vi "EI1050 Read.vi"(8 "error in":errorcluster, 10 "Enable Channel (or -1)":i32=3, 11 "Handle In":i32) -> (0 "error out":errorcluster, 1 "RH [%]":dbl format="%.6f", 2 "Temp [degC]":dbl format="%.6f", 3 "Handle Out":i32, 4 "Temp [degF]":dbl format="%.6f")   [LabVIEW 2021]
panel:
  # "Pass -1 if not using enable/disable."
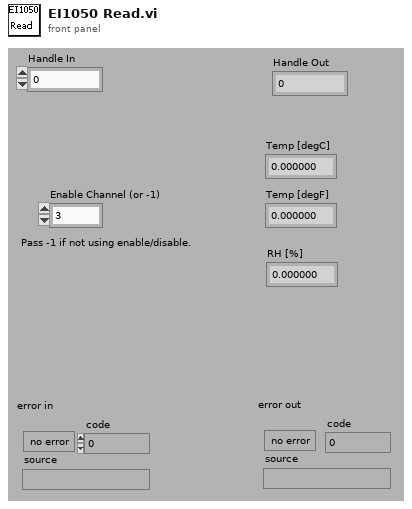
[diagram p1: front panel]
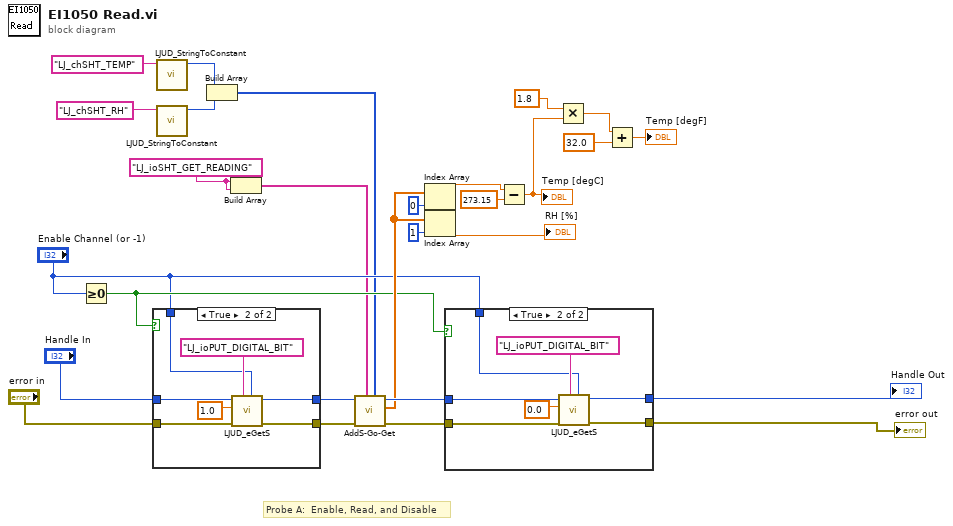
[diagram p0: block diagram]
diagram:
  w12 = "LJ_ioSHT_GET_READING" ("IOType")
  # "Probe A:  Enable, Read, and Disable"
  n1 = Greater Or Equal To 0?(x="Enable Channel (or -1)") -> (x >= 0?=w16:bool)
  n2 = case shown="True" w16 {
    tunnel: [w29 w37] -> w26
    tunnel: [w30 w36] -> w25
    tunnel: "error in" -> [w29 w33]
    tunnel: "Handle In" -> [w30 w32]
    tunnel: "Enable Channel (or -1)" -> [_ w31]
    frame False {
    }
    frame True {
      n3 = call "LJUD_eGetS.vi"("Channel"=w31, "IOType"="LJ_ioPUT_DIGITAL_BIT", "error in"=w33, "Value Write"=1.0, "Handle In"=w32) -> ("error out"=w37:errorcluster, "Handle Out"=w36:i32)  [unwired: 4 in, 1 out]
    }
  }
  n4 = call "LJUD_StringToConstant.vi"("String"="LJ_chSHT_TEMP") -> ("Constant Number"=w11:i32)  [unwired: 9 in, 1 out]
  n5 = call "LJUD_StringToConstant.vi"("String"="LJ_chSHT_RH") -> ("Constant Number"=w10:i32)  [unwired: 9 in, 1 out]
  n6 = Build Array(w11, w10) -> (w6:i32[])
  n7 = Build Array(w12, w12) -> (w7:string[])
  n8 = call "AddS-Go-Get.vi"("Channels"=w6, "IOTypes"=w7, "error in"=w26, "Handle In"=w25) -> ("error out"=w28:errorcluster, "Values Read"=w22:dbl[], "Handle Out"=w27:i32)  [unwired: 5 in]
  n9 = Index Array(array=w22, index=0 ("Index")) -> (element=w24:dbl)
  n10 = Index Array(array=w22, index=1 ("Index")) -> (element=→"RH [%]":dbl)
  n11 = case shown="True" w16 {
    tunnel: w28 -> [w38 w46]
    tunnel: w27 -> [w39 w45]
    tunnel: "Enable Channel (or -1)" -> [_ w42]
    tunnel: [w38 w41] -> w14
    tunnel: [w39 w40] -> w13
    frame False {
    }
    frame True {
      n12 = call "LJUD_eGetS.vi"("Channel"=w42, "IOType"="LJ_ioPUT_DIGITAL_BIT", "error in"=w46, "Value Write"=0.0, "Handle In"=w45) -> ("error out"=w41:errorcluster, "Handle Out"=w40:i32)  [unwired: 4 in, 1 out]
    }
  }
  "error out" <- w14
  "Handle Out" <- w13
  n13 = Subtract(x=w24, y=273.15) -> (x-y=w2:dbl)
  "Temp [degC]" <- w2
  n14 = Multiply(x=1.8, y=w2) -> (x*y=w5:dbl)
  n15 = Add(x=w5, y=32.0) -> (x+y=→"Temp [degF]":dbl)
